vi "Read U8.vi"(11 "Event in":refnum<class "Event U8.lvclass">) -> (2 "U8":u8, 3 "Event out":refnum<class "Event U8.lvclass">)   [LabVIEW 2016, in "Event Actors.lvlib" / "Event U8.lvclass"]
uses:
  Event U8.lvclass
  Event U8.lvclass/Event U8.ctl
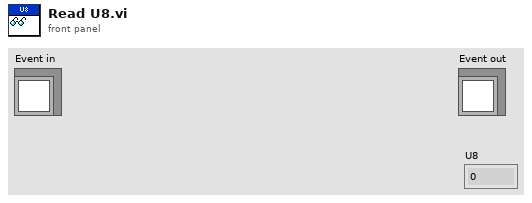
[diagram p1: front panel]
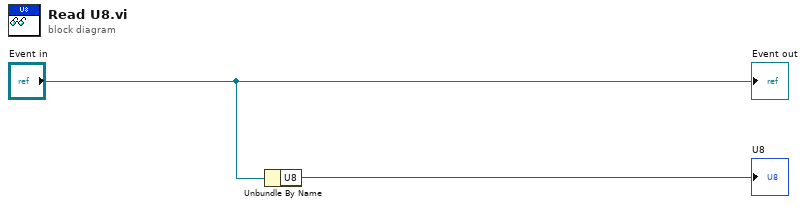
[diagram p0: block diagram]
diagram:
  n1 = Unbundle By Name("Event in") -> ("U8"=→"U8":u8)
  "Event out" <- "Event in"
